vi "Enqueue_Element_Con.vi"(6 "Prioritize?":bool, 8 "error in (no error)":errorcluster, 9 "Data":variant, 10 "State":T1, 11 "Queue in":refnum<queue>) -> (0 "error out":errorcluster)   [LabVIEW 2023]
doc: "This VI enqueues the elements if prioritize is true it puts the elemtns on opposite end"
uses:
  Controls/State.ctl
  Controls/Queued_Data.ctl
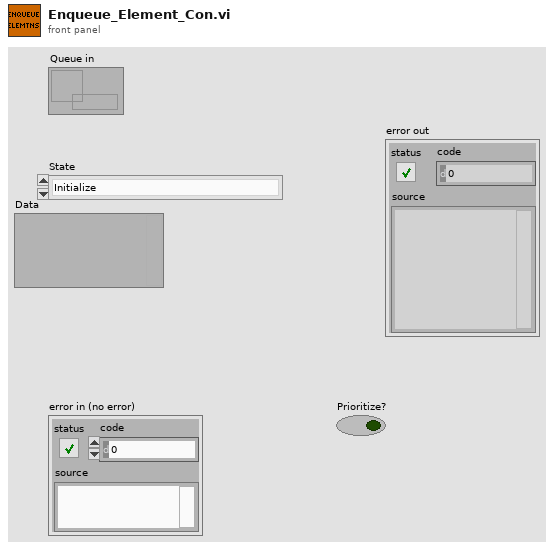
[diagram p1: front panel]
types:
  T1 = typedef "State.ctl" = enum16{"Initialize", "Wait for Something", "Step Completed", "Save Wash Options", "Start Process", "Car Position", "Order Steps to follow", "Underbody Wash", "Bug Remover", "Pre-Soak", "High Pressure Wash", "Low Pressure Wax", "Spot Free Rinse", "Tire Shine Foam", "Air Dry", "Vehicle out of position", "Process Complete", "Stop Application"}
  T2 = typedef "Queued_Data.ctl" = cluster{"State":T1, "Data":variant}
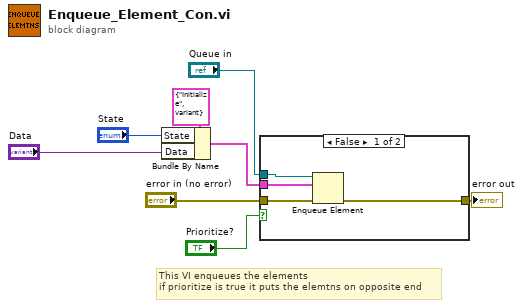
[diagram p0: block diagram]
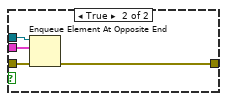
[diagram p2: hidden frame]
diagram:
  # "This VI enqueues the elements\nif prioritize is true it puts the elemtns on opposite end"
  n1 = Bundle By Name(cluster=T2 {"State"=enum."Initialize", "Data"=variant}, "State"="State", "Data"="Data") -> (w7:T2)
  n2 = case shown="False" "Prioritize?" {
    tunnel: w7 -> [w12 w13]
    tunnel: [w11 w15] -> w6
    tunnel: "error in (no error)" -> [w10 w16]
    tunnel: "Queue in" -> [w9 w14]
    frame False {
      n3 = Enqueue Element(queue=w9, element=w12, error in (no error)=w10) -> (error out=w11:errorcluster)  [unwired: 1 in, 2 out]
    }
    frame True {
      n4 = Enqueue Element At Opposite End(queue=w14, element=w13, error in (no error)=w16) -> (error out=w15:errorcluster)  [unwired: 1 in, 2 out]
    }
  }
  "error out" <- w6
